vi "Timing Calculator.vi"(8 "Scan settings array":T1[](array[typedef]) {"No. of EQE scans" min=1.0 step=1.0; "No. of white bias steps" min=1.0 step=1.0; "No. of t const. steps" min=1.0 step=1.0; "Time Constant max (s)" items=["0.01s", "0.03s", "0.1s", "0.3s", "1s", "3s"]; "No. of freq. steps" min=1.0 step=1.0; "J-t Illumination conditions" items=["Light only", "Dark only", "Light then dark", "Dark then light"]; "No. of scan rate steps" min=1.0 step=1.0; "Illumination conditions" items=["Light only", "Dark only", "Light then dark", "Dark then light", "Light then dark then light", "Dark then light then dark"]; "Time Constant min (s)" items=["0.01s", "0.03s", "0.1s", "0.3s", "1s", "3s"]; "Only repeat for best pixel" items=["only for best pixel", "for best 2 pixels", "for best 3 pixels", "for best 4 pixels", "for best 5 pixels", "for best 6 pixels", "for best 7 pixels", "for all pixels"]; "No. of repeat scans" min=1.0 step=1.0; "EQE best pixel only" items=["only the best pixel", "the best 2 pixel", "the best 3 pixel", "the best 4 pixel", "the best 5 pixel", "the best 6 pixel", "the best 7 pixel", "all pixels"]; "P dep best pixel only" items=["only the best pixel", "the best 2 pixels", "the best 3 pixels", "the best 4 pixels", "the best 5 pixels", "the best 6 pixels", "the best 7 pixels", "all pixels"]; "Max power best pixel only" items=["only the best pixel", "the best 2 pixels", "the best 3 pixels", "the best 4 pixels", "the best 5 pixels", "the best 6 pixels", "the best 7 pixels", "all pixels"]; "J-t best pixel only" items=["only the best pixel", "the best 2 pixels", "the best 3 pixels", "the best 4 pixels", "the best 5 pixels", "the best 6 pixels", "the best 7 pixels", "all pixels"]; "Integration time" items=["Fast", "Normal", "High Accuracy"]; "Stabilisation mode" items=["V", "I"]; "Measurement delay (ms)" min=10.0}, 10 "Calibration?":bool, 11 "Measurement queue":T3(array[cluster]) {"Pixel to measure" items=["All", "1", "2", "3", "4", "5", "6", "7", "8"]}) -> (3 "Experiment time (s)":dbl)   [LabVIEW 2011]
uses:
  TypeDefs/Scan settings.ctl
  TypeDefs/Settings Boolean.ctl
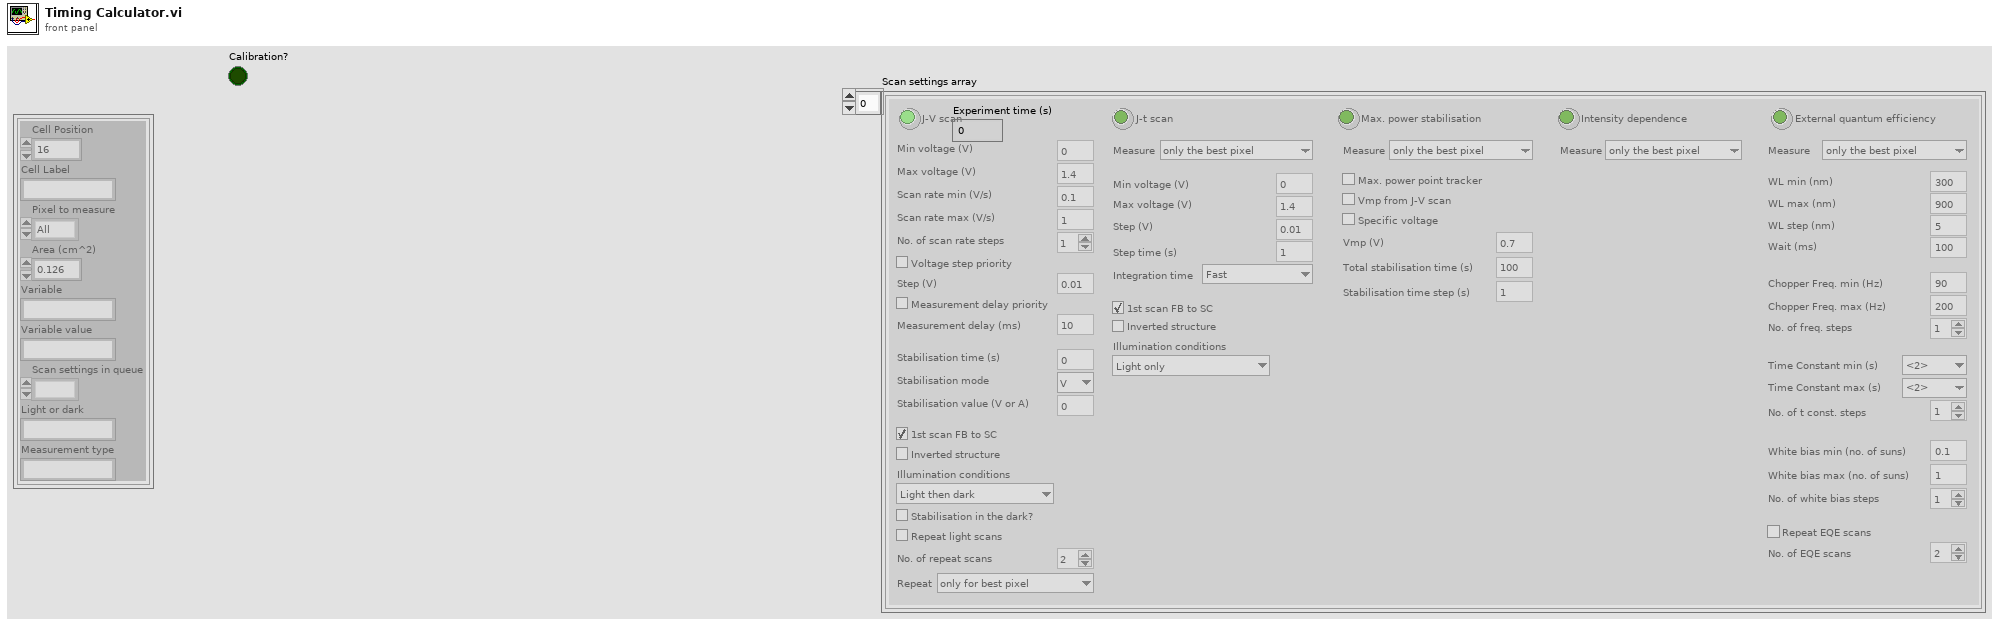
[diagram p1: front panel]
types:
  T1 = typedef "Scan settings.ctl" = cluster{"J-V scan":T2, "J-t scan":bool, "Min voltage (V)":dbl, "Max voltage (V)":dbl, "Step (V)":dbl, "Measurement delay (ms)":dbl, "1st scan FB-SC":bool, "Inverted structure":bool, "Stabilisation time (s)":dbl, "Stabilisation mode":u16, "Stabilisation value (V or A) ":dbl, "Step time (s)":dbl, "Integration time":u16, "Repeat light scans":bool, "Stabilisation in the dark?":bool, "J-t Min (V)":dbl, "J-t Max (V)":dbl, "J-t Step (V)":dbl, "Max. power stabilisation":bool, "J-t 1st scan FB-SC":bool, "J-t Inverted structure":bool, "Max power tracking":bool, "Vmp (V)":dbl, "Total stabilisation time (s)":dbl, "J-t best pixel only":u16, "Max power best pixel only":u16, "Vmp from J-V scan":bool, "Intensity dependence":bool, "P dep best pixel only":u16, "External quantum efficiency":bool, "EQE best pixel only":u16, "WL min (nm)":dbl, "WL max (nm)":dbl, "WL step (nm)":dbl, "Wait (ms)":dbl, "No. of repeat scans":dbl, "Only repeat for best pixel":u16, "Chopper Freq. min (Hz)":dbl, "Time Constant min (s)":dbl, "Stabilisation time step (s)":dbl, "Illumination conditions":u16, "Scan rate min (V/s)":dbl, "Scan rate max (V/s)":dbl, "No. of scan rate steps":dbl, "Scan rate voltage step priority":bool, "Scan rate measurement delay priority":bool, "J-t Illumination conditions":u16, "Chopper Freq. max (Hz)":dbl, "No. of freq. steps":dbl, "Time Constant max (s)":dbl, "No. of t const. steps":dbl, "White bias min (no. of suns)":dbl, "White bias max (no. of suns)":dbl, "No. of white bias steps":dbl, "Repeat EQE scans":bool, "No. of EQE scans":dbl, "Max P stab. Specific voltage":bool}
  T2 = typedef "Settings Boolean.ctl" = bool
  T3 = cluster{"Cell Position":i32, "Cell Label":string, "Pixel to measure":u16, "Area (cm^2)":dbl, "Variable":string, "Variable value":string, "Scan settings in queue":u16, "Light or dark":string, "Measurement type":string}[]
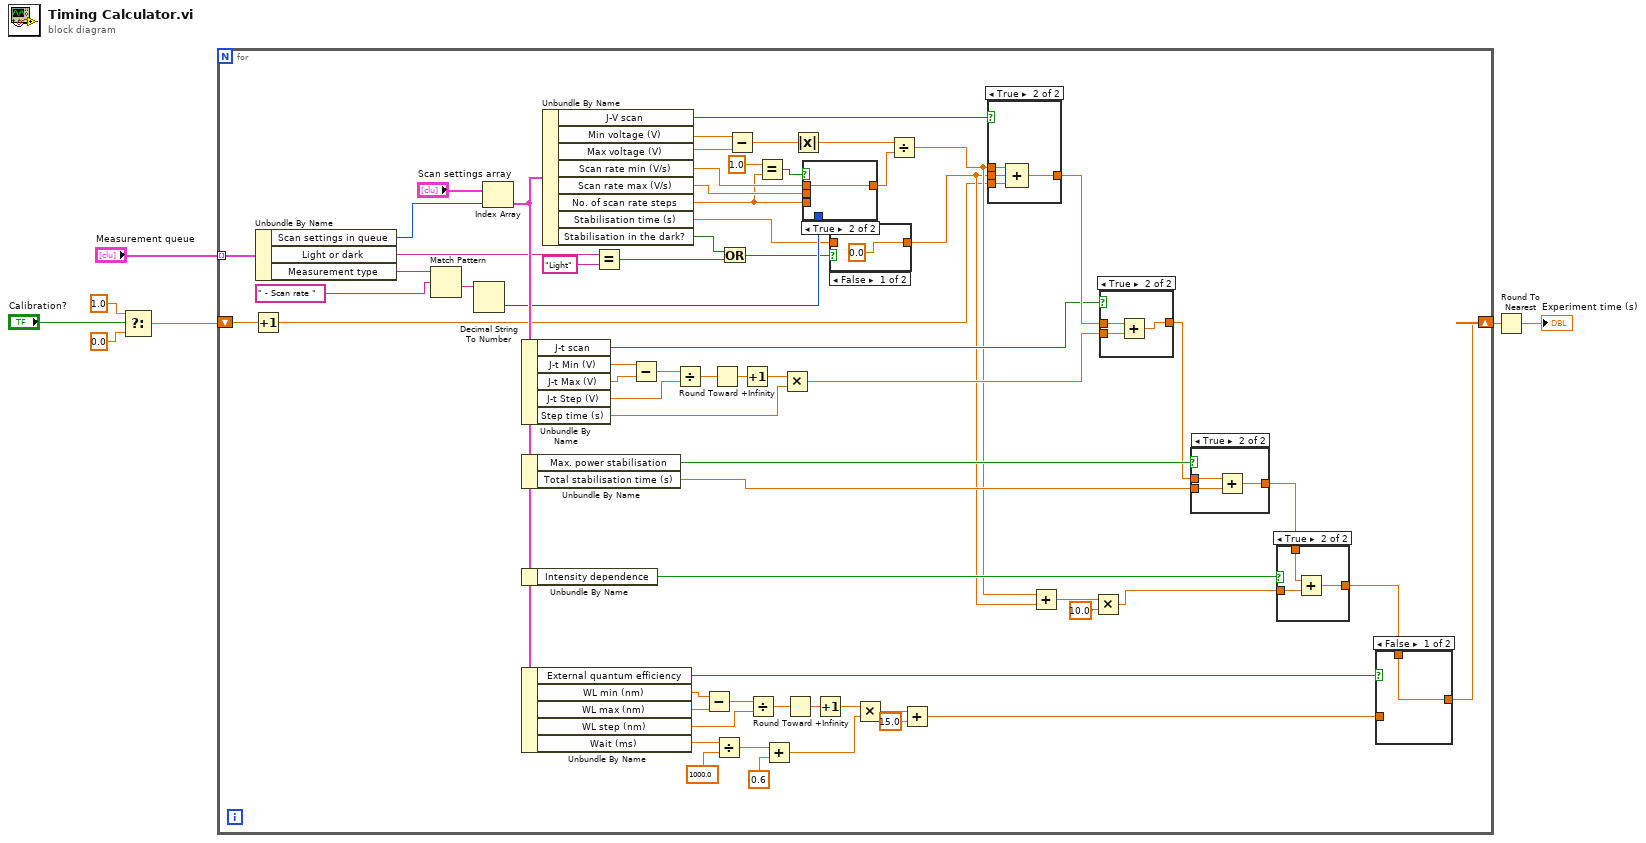
[diagram p0: block diagram]
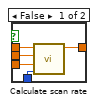
[diagram p3: hidden frame]
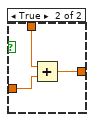
[diagram p4: hidden frame]
diagram:
  n1 = Select(t=1.0, s="Calibration?", f=0.0) -> (s? t:f=w3:dbl)
  n2 = for {
    tunnel: "Measurement queue" -> [w73] mode=indexing
    shift-right: [w31] -> w6
    shift-left: w3 -> [w9]
    n3 = Increment(x=w9) -> (x+1=w8:dbl)
    n4 = Unbundle By Name(w73) -> ("Scan settings in queue"=w71:u16, "Light or dark"=w18:string, "Measurement type"=w19:string)
    n5 = Match Pattern(string=w19, regular expression=" - Scan rate ") -> (after substring=w28:string)  [unwired: 1 in, 3 out]
    n6 = Decimal String To Number(string=w28) -> (number=w27:i32)  [unwired: 2 in, 1 out]
    n7 = Index Array(array="Scan settings array", index=w71) -> (element=w66:T1)
    n8 = Unbundle By Name(w66) -> ("J-t scan"=w55:bool, "J-t Min (V)"=w65:dbl, "J-t Max (V)"=w64:dbl, "J-t Step (V)"=w62:dbl, "Step time (s)"=w58:dbl)
    n9 = Unbundle By Name(w66) -> ("Max. power stabilisation"=w56:bool, "Total stabilisation time (s)"=w53:dbl)
    n10 = Unbundle By Name(w66) -> ("Intensity dependence"=w52:bool)
    n11 = Unbundle By Name(w66) -> ("External quantum efficiency"=w48:bool, "WL min (nm)"=w43:dbl, "WL max (nm)"=w42:dbl, "WL step (nm)"=w41:dbl, "Wait (ms)"=w39:dbl)
    n12 = Unbundle By Name(w66) -> ("J-V scan"=w68:T2, "Min voltage (V)"=w70:dbl, "Max voltage (V)"=w69:dbl, "Scan rate min (V/s)"=w25:dbl, "Scan rate max (V/s)"=w26:dbl, "No. of scan rate steps"=w23:dbl, "Stabilisation time (s)"=w16:dbl, "Stabilisation in the dark?"=w15:bool)
    n13 = Equal?(x=w18, y="Light") -> (x = y?=w13:bool)
    n14 = Subtract(x=w65, y=w64) -> (x-y=w63:dbl)
    n15 = Divide(x=w63, y=w62) -> (x/y=w61:dbl)
    n16 = Subtract(x=w43, y=w42) -> (x-y=w47:dbl)
    n17 = Round Toward +Infinity(x=w61) -> (ceil(x): smallest int >= x=w60:dbl)
    n18 = Divide(x=w39, y=1000.0) -> (x/y=w37:dbl)
    n19 = Or(x=w15, y=w13) -> (x .or. y?=w14:bool)
    n20 = Subtract(x=w70, y=w69) -> (x-y=w30:dbl)
    n21 = Increment(x=w60) -> (x+1=w59:dbl)
    n22 = Divide(x=w47, y=w41) -> (x/y=w46:dbl)
    n23 = Equal?(x=1.0 ("y"), y=w23) -> (x = y?=w22:bool)
    n24 = Add(x=w37, y=0.6) -> (x+y=w36:dbl)
    n25 = Multiply(x=w59, y=w58) -> (x*y=w57:dbl)
    n26 = Round Toward +Infinity(x=w46) -> (ceil(x): smallest int >= x=w45:dbl)
    n27 = Absolute Value(x=w30) -> (abs(x)=w21:dbl)
    n28 = case shown="True" w22 {
      tunnel: w27 -> [w80 _]
      tunnel: w23 -> [w79 _]
      tunnel: w26 -> [w78 _]
      tunnel: w25 -> [w77 w81]
      tunnel: [w76 w81] -> w20
      frame False {
        n29 = call "Calculate scan rate.vi"("Scan rate number"=w80, "Number of steps"=w79, "Scan rate max (V/s)"=w78, "Scan rate min (V/s)"=w77) -> ("Scan rate"=w76:dbl)  [unwired: 7 in]
      }
      frame True {
      }
    }
    n30 = Increment(x=w45) -> (x+1=w44:dbl)
    n31 = case shown="False" w14 {
      tunnel: w16 -> [_ w75]
      tunnel: [0.0 ("Stabilisation time (s)") w75] -> w10
      frame False {
      }
      frame True {
      }
    }
    n32 = Multiply(x=w44, y=w36) -> (x*y=w34:dbl)
    n33 = Divide(x=w21, y=w20) -> (x/y=w11:dbl)
    n34 = Add(x=w34, y=15.0) -> (x+y=w32:dbl)
    n35 = case shown="True" w68 {
      tunnel: w11 -> [_ w102]
      tunnel: [w98 w101] -> w67
      tunnel: w8 -> [w98 w100]
      tunnel: w10 -> [_ w99]
      frame False {
      }
      frame True {
        n36 = Compound Arithmetic op=ADD(w102, w99, w100) -> (w101:dbl)
      }
    }
    n37 = Add(x=w11, y=w10) -> (x+y=w12:dbl)
    n38 = Multiply(x=w12, y=10.0) -> (x*y=w49:dbl)
    n39 = case shown="True" w55 {
      tunnel: w67 -> [w94 w97]
      tunnel: w57 -> [_ w96]
      tunnel: [w94 w95] -> w54
      frame False {
      }
      frame True {
        n40 = Add(x=w97, y=w96) -> (x+y=w95:dbl)
      }
    }
    n41 = case shown="True" w56 {
      tunnel: w54 -> [w90 w93]
      tunnel: w53 -> [_ w92]
      tunnel: [w90 w91] -> w50
      frame False {
      }
      frame True {
        n42 = Add(x=w93, y=w92) -> (x+y=w91:dbl)
      }
    }
    n43 = case shown="True" w52 {
      tunnel: w50 -> [w86 w89]
      tunnel: w49 -> [_ w88]
      tunnel: [w86 w87] -> w35
      frame False {
      }
      frame True {
        n44 = Add(x=w89, y=w88) -> (x+y=w87:dbl)
      }
    }
    n45 = case shown="False" w48 {
      tunnel: w35 -> [w82 w85]
      tunnel: w32 -> [_ w84]
      tunnel: [w82 w83] -> w31
      frame False {
      }
      frame True {
        n46 = Add(x=w85, y=w84) -> (x+y=w83:dbl)
      }
    }
  }
  n47 = Round To Nearest(number=w6) -> (nearest integer value=→"Experiment time (s)":dbl)
